vi "Stop Core.vi"(10 "final error code":i32, 11 "SpectrumAnalyzerUI in":refnum<class "SpectrumAnalyzerUI.lvclass">) -> (3 "SpectrumAnalyzerUI out":refnum<class "SpectrumAnalyzerUI.lvclass">)   [LabVIEW 2023, in "SpectrumAnalyzerUI.lvlib" / "SpectrumAnalyzerUI.lvclass"]
doc: "(<B>Filename</B>: Actor Framework.lvlib:Actor.lvclass:Stop Core.vi)\n\nDefines what the actor does before it stops. Use the <B>final error code</B> input to determine whether the actor shut down in response to an error.\n\nBy default, this method passes the Stop message along to all auto-stop nested actors. A descendant class may override this method to define additional behavior, such as shutting down any processes the actor initiated in its override of the Actor Core method."
uses:
  SpectrumAnalyzerUI.lvclass
  SpectrumAnalyzerUI.lvclass/SpectrumAnalyzerUI.ctl
  <vilib>/ActorFramework/Actor/Actor.lvclass
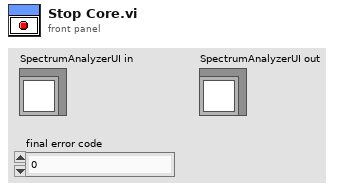
[diagram p1: front panel]
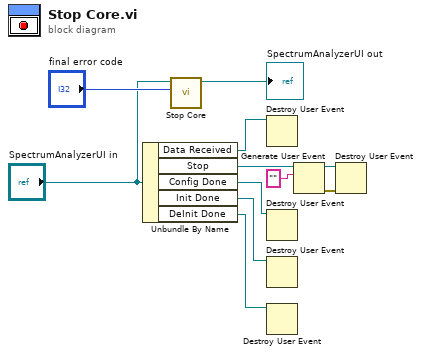
[diagram p0: block diagram]
diagram:
  n1 = Unbundle By Name("SpectrumAnalyzerUI in") -> ("Data Received"=w4:refnum<user-event>, "Stop"=w8:refnum<user-event>, "Config Done"=w2:refnum<user-event>, "Init Done"=w1:refnum<user-event>, "DeInit Done"=w3:refnum<user-event>)
  n2 = call-parent "Stop Core.vi"("final error code"="final error code", "Actor in"="SpectrumAnalyzerUI in") -> ("Actor out"=→"SpectrumAnalyzerUI out":refnum<class "SpectrumAnalyzerUI.lvclass">)  [unwired: 9 in]
  n3 = Destroy User Event(user event=w4) -> ()  [unwired: 1 in, 1 out]
  n4 = Destroy User Event(user event=w2) -> ()  [unwired: 1 in, 1 out]
  n5 = Destroy User Event(user event=w1) -> ()  [unwired: 1 in, 1 out]
  n6 = Destroy User Event(user event=w3) -> ()  [unwired: 1 in, 1 out]
  n7 = Generate User Event(user event=w8, event data cluster="" ("event data")) -> (user event out=w7:refnum<user-event>, error out=w6:errorcluster)  [unwired: 2 in]
  n8 = Destroy User Event(user event=w7, error in=w6) -> ()  [unwired: 1 out]
